vi "RSZVB Set Internal Signal Source.vi"(8 "error in (no error)":errorcluster {"code" format="%.0x"}, 9 "Internal Signal Source (0)":i32, 10 "Channel (1)":i32=1, 11 "VISA session":refnum<visa-resource-name>) -> (0 "error out":errorcluster {"code" format="%.0x"}, 3 "dup VISA session":refnum<visa-resource-name>)   [LabVIEW 2011]
doc: "This VI sets an analyzer port as a signal source for the LO signal (internal source).\n\nRemote-control command(s):\n[SENSe<Ch>:]FREQuency:CONVersion:MIXer:LOINternal NONE | <port_number>"
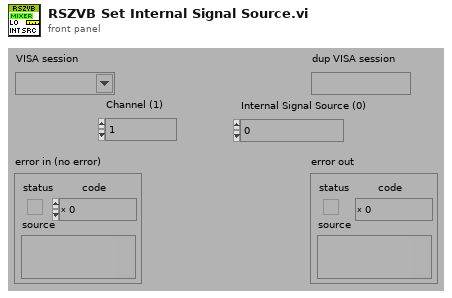
[diagram p1: front panel]
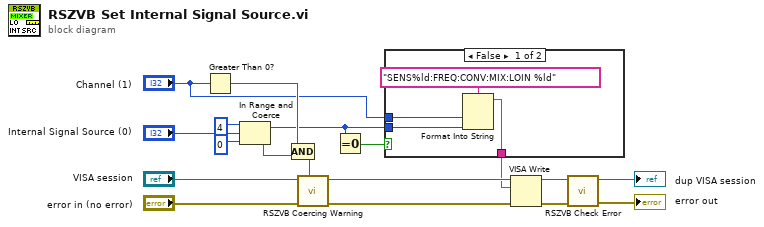
[diagram p0: block diagram]
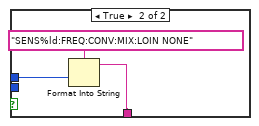
[diagram p2: hidden frame]
diagram:
  n1 = Greater Than 0?(x="Channel (1)") -> (x > 0?=w11:bool)
  n2 = In Range and Coerce(upper limit=4, x="Internal Signal Source (0)", lower limit=0) -> (coerced(x)=w2:i32, In Range?=w12:bool)
  n3 = Compound Arithmetic op=AND(w11, w12) -> (w10:bool)
  n4 = call "RSZVB Coercing Warning.vi"("In Range?"=w10, "error in (no error)"="error in (no error)", "VISA session"="VISA session") -> ("error out"=w15:errorcluster, "dup VISA session"=w16:refnum<visa-resource-name>)  [unwired: 7 in]
  n5 = Equal To 0?(x=w2) -> (x = 0?=w1:bool)
  n6 = case shown="False" w1 {
    tunnel: [w21 w23] -> w9
    tunnel: "Channel (1)" -> [w20 w24]
    tunnel: w2 -> [w19 _]
    frame False {
      n7 = Format Into String(format string="SENS%ld:FREQ:CONV:MIX:LOIN %ld", w20, w19) -> (resulting string=w21:string)  [unwired: 2 in, 1 out]
    }
    frame True {
      n8 = Format Into String(format string="SENS%ld:FREQ:CONV:MIX:LOIN NONE", w24) -> (resulting string=w23:string)  [unwired: 2 in, 1 out]
    }
  }
  n9 = VISA Write(VISA resource name=w16, write buffer=w9, error in (no error)=w15) -> (VISA resource name out=w13:refnum<visa-resource-name>, error out=w14:errorcluster)  [unwired: 1 out]
  n10 = call "RSZVB Check Error.vi"("error in (no error)"=w14, "VISA session"=w13) -> ("error out"=→"error out":errorcluster, "dup VISA session"=→"dup VISA session":refnum<visa-resource-name>)  [unwired: 8 in]
